vi "Actor Async.vi"(5 "API Q":refnum<queue>, 7 "Error Q":refnum<queue>, 9 "Wait Core":bool, 10 "Caller Queue":refnum<class "Priority Message Queue.lvclass">, 11 "Actor in":refnum<class "Actor.lvclass">) -> ()   [LabVIEW 2022 SP3, in "Artifex.lvlib" / "Actor.lvclass"]
uses:
  Actor.lvclass
  Actor Proxy/Actor API.lvclass
  Priority Message Queue/Priority Message Queue.lvclass
  Message/Message.lvclass
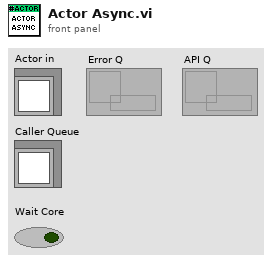
[diagram p1: front panel]
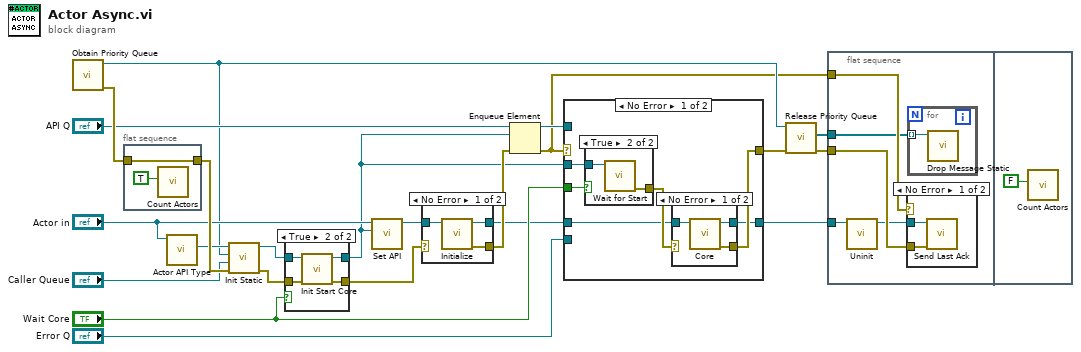
[diagram p0: block diagram]
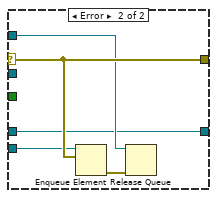
[diagram p5: hidden frame]
diagram:
  n1 = call "Obtain Priority Queue.vi"() -> ("error out"=w21:errorcluster, "Priority Message Queue out"=w5:refnum<class "Priority Message Queue.lvclass">)  [unwired: 10 in]
  n2 = flat-sequence {
    tunnel: w21 -> [w23]
    tunnel: [w23] -> w22
    frame #0 {
      n3 = call "Count Actors.vi"("Increment"=TRUE) -> ()  [unwired: 11 in]
    }
  }
  n4 = call-dynamic "Actor API Type.vi"("Actor in"="Actor in") -> ("Actor API Type"=w20:refnum<class "Actor API.lvclass">)  [unwired: 10 in]
  n5 = call "Init Static.vi"("error in (no error)"=w22, "Caller Queue"="Caller Queue", "Self Queue"=w5, "Actor API in"=w20) -> ("error out"=w19:errorcluster, "Actor API out"=w18:refnum<class "Actor API.lvclass">)  [unwired: 6 in]
  n6 = case shown="True" "Wait Core" {
    tunnel: w19 -> [w25 w29]
    tunnel: w18 -> [w26 w30]
    tunnel: [w26 w28] -> w8
    tunnel: [w25 w27] -> w14
    frame False {
    }
    frame True {
      n7 = call "Init Start Core.vi"("error in (no error)"=w29, "Actor API in"=w30) -> ("error out"=w27:errorcluster, "Actor API out"=w28:refnum<class "Actor API.lvclass">)  [unwired: 8 in]
    }
  }
  n8 = call-dynamic "Set API.vi"("Actor API"=w8, "Actor in"="Actor in") -> ("Actor out"=w15:refnum<class "Actor.lvclass">)  [unwired: 8 in, 1 out]
  n9 = case shown="No Error" w14 {
    selector: w14 -> [_ w35]
    tunnel: w15 -> [w33 w34]
    tunnel: [w32 w35] -> w12
    tunnel: [w31 w34] -> w7
    frame No Error {
      n10 = call-dynamic "Initialize.vi"("Actor in"=w33) -> ("error out"=w32:errorcluster, "Actor out"=w31:refnum<class "Actor.lvclass">)  [unwired: 9 in]
    }
    frame Error {
    }
  }
  n11 = Enqueue Element(queue="API Q", element=w8, error in (no error)=w12) -> (queue out=w10:refnum<queue>, error out=w2:errorcluster)  [unwired: 1 in, 1 out]
  n12 = case shown="No Error" w2 {
    selector: w2 -> [_ w53]
    tunnel: "Error Q" -> [_ w52]
    tunnel: w10 -> [_ w50]
    tunnel: [w37 w53] -> w6
    tunnel: "Wait Core" -> [w40 _]
    tunnel: w8 -> [w39 _]
    tunnel: w7 -> [w38 w49]
    tunnel: [w36 w49] -> w4
    frame No Error {
      n13 = case shown="True" w40 {
        tunnel: w39 -> [_ w48]
        tunnel: [_ w47] -> w41
        frame False {
        }
        frame True {
          n14 = call "Wait for Start.vi"("Actor API in"=w48) -> ("error out"=w47:errorcluster)  [unwired: 9 in, 1 out]
        }
      }
      n15 = case shown="No Error" w41 {
        selector: w41 -> [_ w46]
        tunnel: w38 -> [w44 w45]
        tunnel: [w43 w46] -> w37
        tunnel: [w42 w45] -> w36
        frame No Error {
          n16 = call-dynamic "Core.vi"("Actor in"=w44) -> ("error out"=w43:errorcluster, "Actor out"=w42:refnum<class "Actor.lvclass">)  [unwired: 9 in]
        }
        frame Error {
        }
      }
    }
    frame Error {
      n17 = Enqueue Element(queue=w52, element=w53) -> (error out=w51:errorcluster)  [unwired: 2 in, 2 out]
      n18 = Release Queue(queue=w50, error in (no error)=w51) -> ()  [unwired: 1 in, 3 out]
    }
  }
  n19 = call "Release Priority Queue.vi"("error in (no error)"=w6, "Priority Message Queue in"=w5) -> ("error out"=w3:errorcluster, "Remaining Elements"=w1:refnum<class "Message.lvclass">[])  [unwired: 8 in]
  n20 = flat-sequence {
    tunnel: w4 -> [w57]
    tunnel: w3 -> [w58]
    tunnel: w2 -> [w56]
    tunnel: w1 -> [w54]
    frame #0 {
      n21 = call-dynamic "Uninit.vi"("Actor in"=w57) -> ("Actor out"=w55:refnum<class "Actor.lvclass">)  [unwired: 9 in, 1 out]
      n22 = case shown="No Error" w56 {
        tunnel: w55 -> [w61 _]
        tunnel: w58 -> [w60 _]
        frame No Error {
          n23 = call "Send Last Ack.vi"("error in (no error)"=w60, "Actor in"=w61) -> ()  [unwired: 9 in, 1 out]
        }
        frame Error {
        }
      }
      n24 = for {
        tunnel: w54 -> [w59] mode=indexing
        n25 = call "Drop Message Static.vi"("Message in"=w59) -> ()  [unwired: 11 in]
      }
    }
    frame #1 {
      n26 = call "Count Actors.vi"("Increment"=FALSE) -> ()  [unwired: 11 in]
    }
  }
